vi "toRMS.vi"(11 "Input":dbl) -> (3 "Output [Vrms]":dbl)   [LabVIEW 2019, in "FPGA.lvlib"]
uses:
  FPGA.lvlib
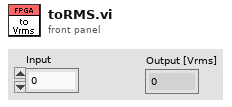
[diagram p1: front panel]
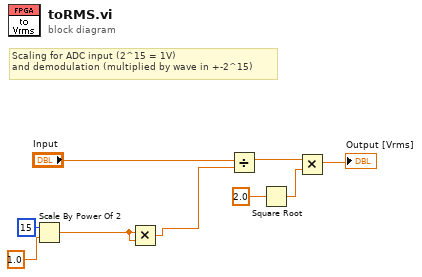
[diagram p0: block diagram]
diagram:
  # "Scaling for ADC input (2^15 = 1V)\nand demodulation (multiplied by wave in +-2^15)"
  n1 = Scale By Power Of 2(n=i16 15, x=1.0) -> (x*2^n=w7:dbl)
  n2 = Multiply(x=w7, y=w7) -> (x*y=w4:dbl)
  n3 = Divide(x="Input", y=w4) -> (x/y=w2:dbl)
  n4 = Square Root(x=2.0) -> (sqrt(x)=w1:dbl)
  n5 = Multiply(x=w2, y=w1) -> (x*y=→"Output [Vrms]":dbl)
